vi "createEdge.vi"(5 "error in (no error)":errorcluster, 6 "node 2":dbl[](array[numeric]), 7 "node1":dbl[](array[numeric]), 8 "Map":T1) -> (0 "error out":errorcluster, 2 "Distance":dbl, 3 "FreePath":bool)   [LabVIEW 2009]
uses:
  <vilib>/Analysis/Matrix/Datatypes/RealMatrix.ctl
  <vilib>/imath/engines/lvmath2/RunTimeEngine/ErrorHandling/NIMS_Finalize Error.vi
  <vilib>/imath/engines/lvmath2/RunTimeEngine/Parser/MC_Version.vi
  <vilib>/imath/engines/lvmath2/RunTimeEngine/NodeEndStatement/NIMS_NodeEndStatement_Output.vi
  <instcachedir>/0/NIMS_NodeEndStatement_Output_B70DDD75627E4997AAE11E9955EDAA25.lvgen/NIMS_NodeEndStatement_Output_B70DDD75627E4997AAE11E9955EDAA25_001.vi
  <instcachedir>/0/NIMS_NodeEndStatement_Output_B70DDD75627E4997AAE11E9955EDAA25.lvgen/NIMS_NodeEndStatement_Output_B70DDD75627E4997AAE11E9955EDAA25_000.vi
  <instcachedir>/0/NIMS_NodeEndStatement_Output_B70DDD75627E4997AAE11E9955EDAA25.lvgen/NIMS_NodeEndStatement_Output_B70DDD75627E4997AAE11E9955EDAA25_005.vi
  <vilib>/imath/engines/lvmath/Functions/Error Handling/MergeErrorsWrapper.vi
  <vilib>/imathl/engines/lvmath/Functions/Error Handling/Create Error.vi
  <vilib>/Analysis/Matrix/Numeric/Conversions/Matrix To Array - RM.vi
  <vilib>/imath/engines/lvmath2/RunTimeEngine/VariableToken/Read/NIMS_Get Elements - RV(_) - Check.vi
  <instcachedir>/0/NIMS_Get Elements - RV(_) - Check_60F12861D0564803969A5D0D0D1716CD.lvgen/NIMS_Get Elements - RV(_) - Check_60F12861D0564803969A5D0D0D1716CD_000.vi
  <vilib>/imath/engines/lvmath2/RunTimeEngine/BuiltInFunctions/abs/NIMS_abs(signed).vi
  <instcachedir>/0/NIMS_abs(signed)_C4FCB8E6058B49B797C7C8D53CA5F6EC.lvgen/NIMS_abs(signed)_C4FCB8E6058B49B797C7C8D53CA5F6EC_000.vi
  <vilib>/imath/engines/lvmath2/RunTimeEngine/BuiltInFunctions/max/2 inputs/NIMS_max(RG,RG)-no size check.vi
  <instcachedir>/0/NIMS_max(RG,RG)-no size check_F871939977644B7683C1350DCCAD7557.lvgen/NIMS_max(RG,RG)-no size check_F871939977644B7683C1350DCCAD7557_000.vi
  <vilib>/imath/engines/lvmath/Functions/Error Handling/error.ctl
  <vilib>/imath/engines/lvmath/Functions/Error Handling/MC_Mask_Errors.vi
  <vilib>/imath/engines/lvmath2/RunTimeEngine/VariableToken/Read/NIMS_Get Elements - SorM(_,_) - Check(_) - Check(_).vi
  <instcachedir>/0/NIMS_Get Elements - SorM(_,_) - Check(_) - Check(_)_765307169EBF4B10AFB614967F0850B3.lvgen/NIMS_Get Elements - SorM(_,_) - Check(_) - Check(_)_765307169EBF4B10AFB614967F0850B3_000.vi
  <vilib>/imath/engines/lvmath2/RunTimeEngine/CommandStatement/MC_CommandStatement_break.vi
  <vilib>/imath/engines/lvmath2/RunTimeEngine/VariableToken/Read/NIMS_Get Elements - V(S).vi
  <instcachedir>/0/NIMS_Get Elements - V(S)_E93C7964B0344523ACA81A64099422EF.lvgen/NIMS_Get Elements - V(S)_E93C7964B0344523ACA81A64099422EF_000.vi
  <vilib>/Analysis/Matrix/NI_Matrix.lvlib
panel:
  out "k":i32
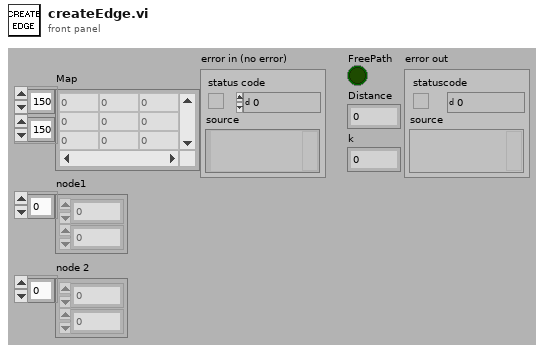
[diagram p1: front panel]
types:
  T1 = typedef "NI_Matrix.lvlib/RealMatrix.ctl" = dbl[][]
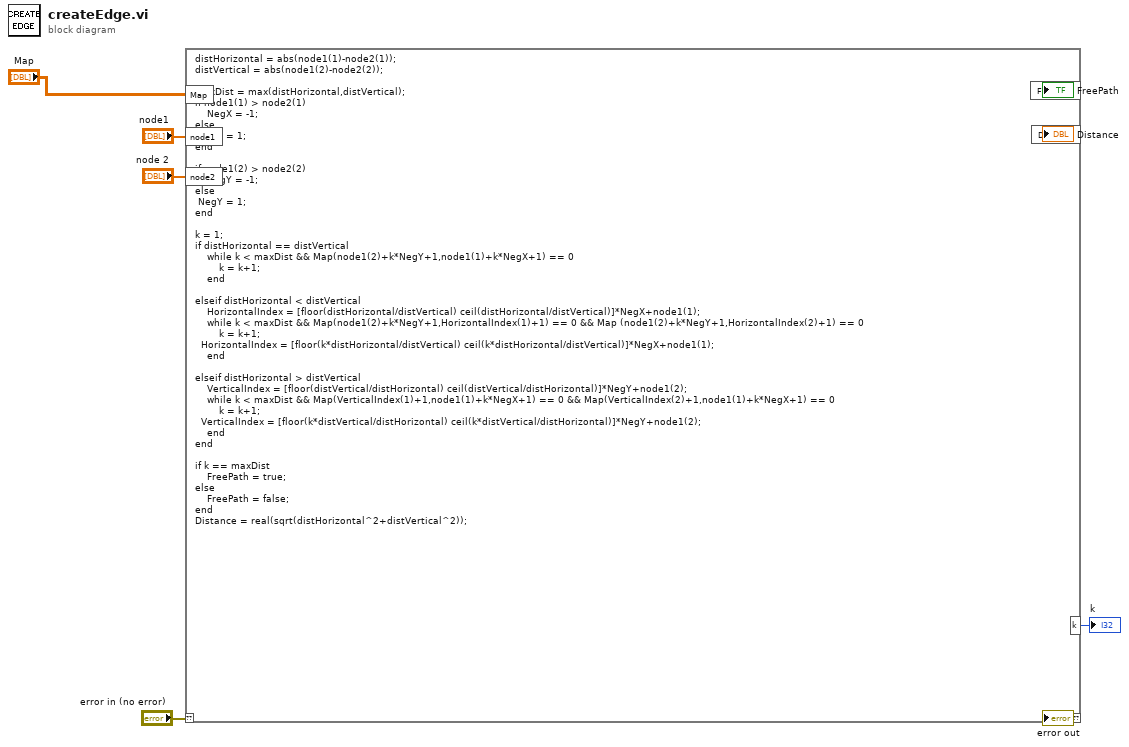
[diagram p0: block diagram]
diagram:
  n1 = mathscript code="distHorizontal = abs(node1(1)-node2(1));\ndistVertical = abs(node1(2)-node2(2));\n\nmaxDist = max(distHorizontal,distVertical);\nif node1(1) > node2(1)\n    NegX = -1;\nelse\n\tNegX = 1;\nend\n\nif node1(2) > node2(2)\n    NegY = -1;\nelse\n\tNegY = 1;\nend\n\nk = 1;\nif distHorizontal == distVertical\n    while k < maxDist && Map(node1(2)+k*NegY+1,node1(1)+k*NegX+1) == 0\n        k = k+1;\n    end\n    \nelseif distHorizontal < distVertical\n    HorizontalIndex = [floor(distHorizontal/distVertical) ceil(distHorizontal/distVertical)]*NegX+node1(1);\n    while k < maxDist && Map(node1(2)+k*NegY+1,HorizontalIndex(1)+1) == 0 && Map (node1(2)+k*NegY+1,HorizontalIndex(2)+1) == 0\n        k = k+1;\n\t\tHorizontalIndex = [floor(k*distHorizontal/distVertical) ceil(k*distHorizontal/distVertical)]*NegX+node1(1);\n    end\n    \nelseif distHorizontal > distVertical\n    VerticalIndex = [floor(distVertical/distHorizontal) ceil(distVertical/distHorizontal)]*NegY+node1(2);\n    while k < maxDist && Map(VerticalIndex(1)+1,node1(1)+k*NegX+1) == 0 && Map(VerticalIndex(2)+1,node1(1)+k*NegX+1) == 0\n        k = k+1;\n\t\tVerticalIndex = [floor(k*distVertical/distHorizontal) ceil(k*distVertical/distHorizontal)]*NegY+node1(2);\n    end\nend\n\nif k == maxDist\n    FreePath = true;\nelse\n    FreePath = false;\nend\nDistance = real(sqrt(distHorizontal^2+distVertical^2));"("??"="error in (no error)", "Map"="Map", "node1"="node1", "node2"="node 2") -> ("??"=→"error out":errorcluster, "FreePath"=→"FreePath":bool, "Distance"=→"Distance":dbl, "k"=→"k":i32)
